vi "Start Water Draw Test Sequence SM.vi"(0 "Degree Setting":dbl=58.0, 1 "Equipment":T3={"COM Port"="COM1", "MW100"="MW100", "AG34970"="A-34972A", "WT500"="WT500"}, 2 "Semiphore":T2, 5 "Flow rate setting":dbl=3.0, 7 "Temp Band(+/- F)":dbl=50.0, 11 "Error In":errorcluster, 12 "Flow Chart Ref":refnum<vi>, 13 "Test Condition":T1(ring)=enum."DRK500,Station1,downspout") -> (4 "Downspout Flow":dbl=3.8899999999999997, 6 "Downspout Temp":dbl=76.8, 8 "Flow rate setting out":dbl=85.11482133995038, 15 "Error Out":errorcluster)   [LabVIEW 2009]
uses:
  EquipReferences.ctl
  Intellifaucet/Intellfaucet Mode.ctl
  ChannelSettings.ctl
panel:
  in  "Purge Min Time":i32=10000
  out "FlowSetTime":dbl
  out "FlowSetStartTime":dbl=3.0
  out "Settle Time Start":dbl format="%.2f"
  out "Purging":i32
  out "FlolwErrors":bool[](array[boolean])
  out "TempErrors":bool[](array[boolean])
  out "TempSet Time (sec)":dbl format="%.2f"
  out "error out":errorcluster
  in  "Sample Period(mS)":u32=500
  in  "Steady State Persist Time(mS)":u32=5000
  in  "Flow Adjust Time (3s)":dbl=3.0
  in  "Flow SettleTimeLimit(S)":dbl=300.0
  out "Downspout Flow Chart":dbl(graph)=3.8899999999999997
  out "Current State":string="Flow Settle"
  out "Downspout Temp Chart":dbl(graph)=76.8
  out "-E":dbl=54.11
  in  "Proportional Control Adjust Rate":dbl=0.1
  in  "Temp SettleTimeLimit(S)":dbl=20.0
  in  "Flow Band (+/-GPM)":dbl=0.25
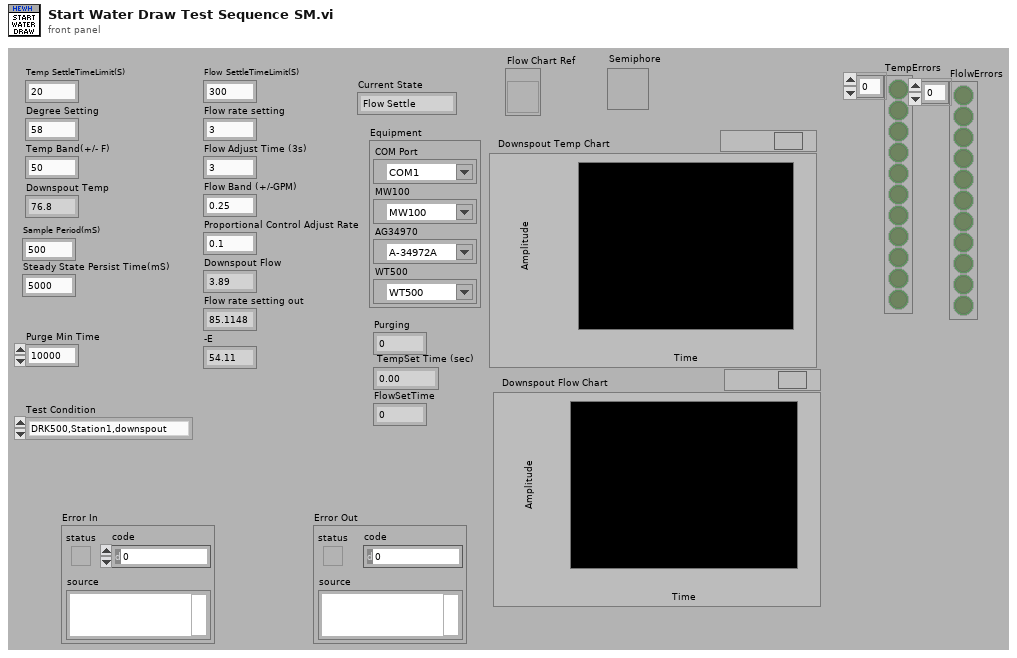
[diagram p1: front panel]
types:
  T1 = enum16{"DRK500,Station1", "DRK375,Lab", "SRK500,Station1,5GPM FR", "DRK500,Station1,downspout"}
  T2 = typedef "Semaphore RefNum" = refnum<k1>
  T3 = typedef "EquipReferences.ctl" = cluster{"COM Port":refnum<visa-resource-name>, "MW100":refnum<visa-resource-name>, "AG34970":refnum<visa-resource-name>, "WT500":refnum<visa-resource-name>}
  T4 = typedef "Intellfaucet Mode.ctl" = enum16{"Adjust Temp", "Adjust Flow", "Start Flow", "Stop Flow"}
  T5 = typedef "ChannelSettings.ctl" = u32
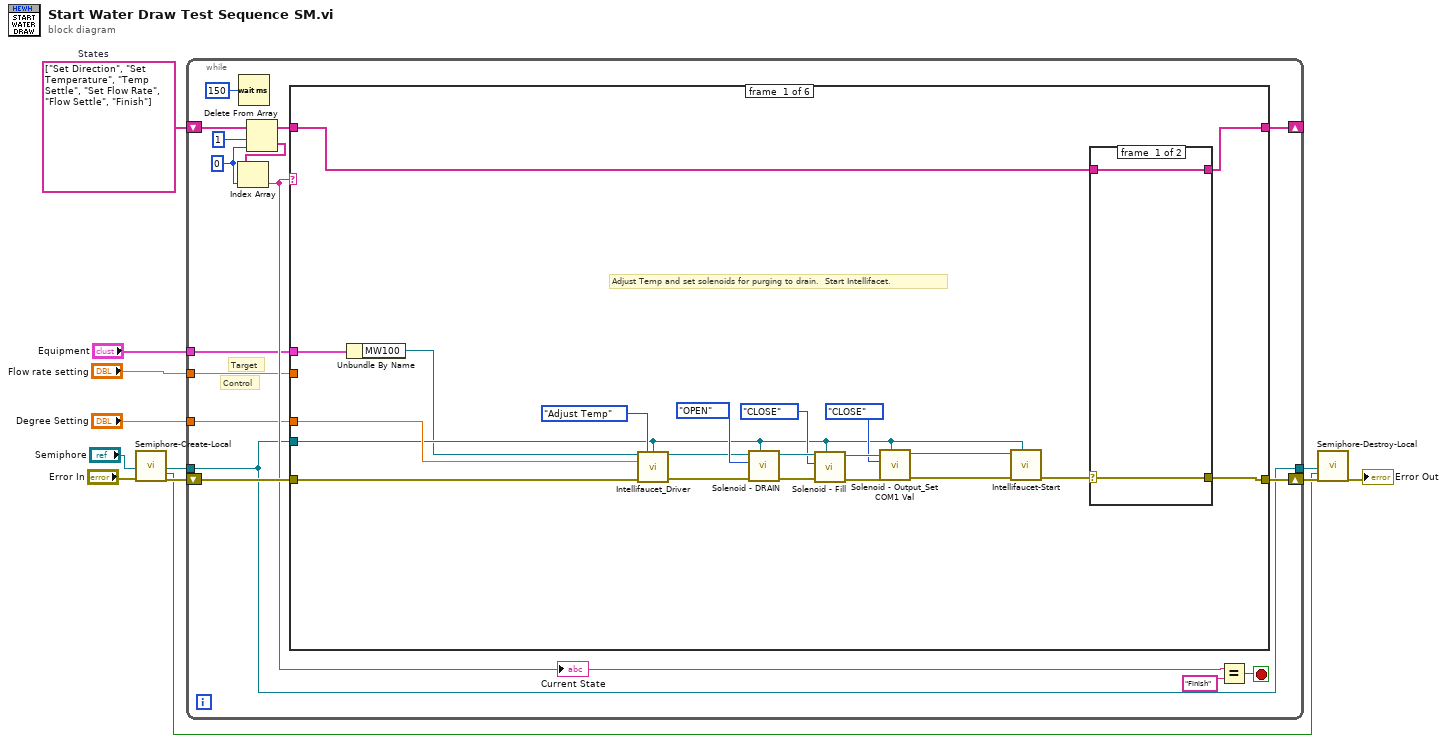
[diagram p0: block diagram]
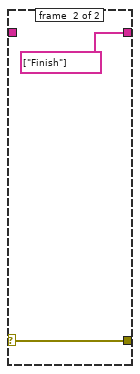
[diagram p2: hidden frame]
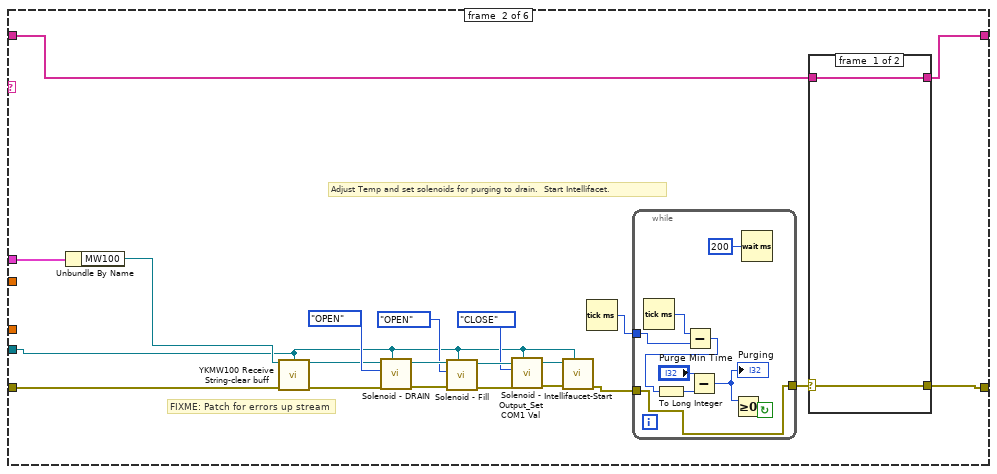
[diagram p3: hidden frame]
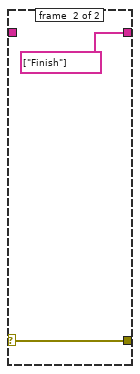
[diagram p4: hidden frame]
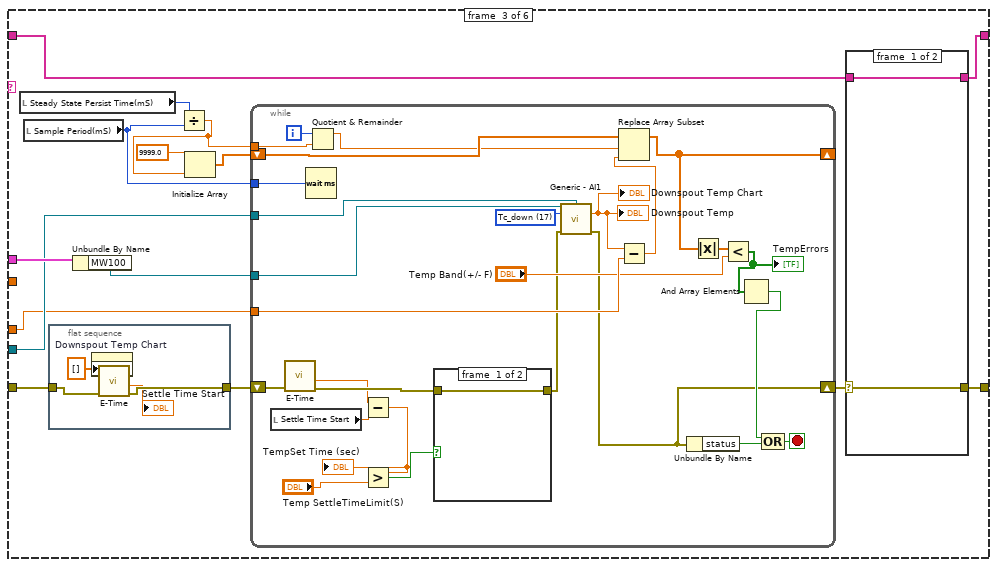
[diagram p5: hidden frame]
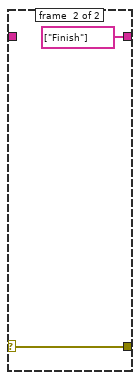
[diagram p6: hidden frame]
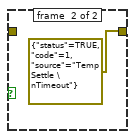
[diagram p7: hidden frame]
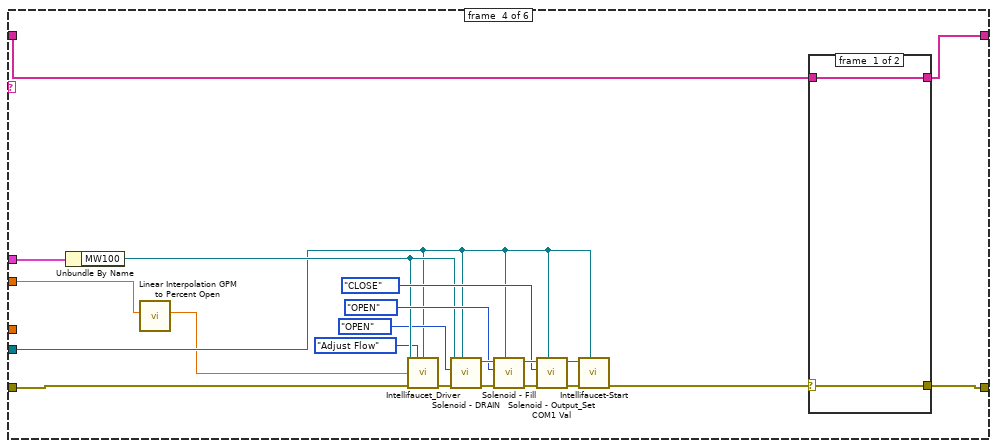
[diagram p8: hidden frame]
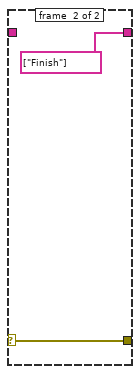
[diagram p9: hidden frame]
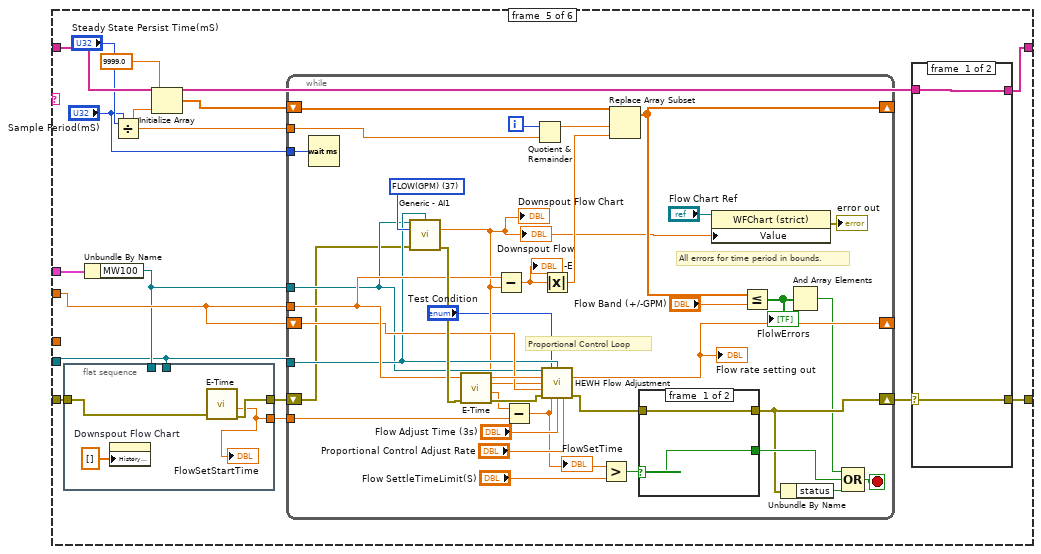
[diagram p10: hidden frame]
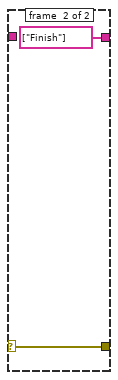
[diagram p11: hidden frame]
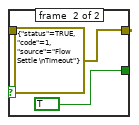
[diagram p12: hidden frame]
diagram:
  w12 = string[] ["Set Direction", "Set Temperature", "Temp Settle", "Set Flow Rate", "Flow Settle", "Finish"]  # States
  n1 = call "Semiphore-Create-Local.vi"("Semiphore"="Semiphore", "error in (no error)"="Error In") -> ("semaphore"=w2:T2, "Local?"=w3:bool, "error out"=w6:errorcluster)  [unwired: 15 in]
  n2 = while {
    shift-right: [w24] -> _
    shift-left: w12 -> [w28]
    shift-right: [w21] -> w5
    shift-left: w6 -> [w20]
    tunnel: "Equipment" -> [w16]
    tunnel: "Degree Setting" -> [w15]
    tunnel: "Flow rate setting" -> [w14]
    tunnel: w2 -> [w13]
    tunnel: [w13] -> w1
    stop <- w19 stop-if-true
    w25 = 0 ("index")
    # "Control"
    # "Target"
    n3 = Wait (ms)(milliseconds to wait=u32 150) -> ()  [unwired: 1 out]
    n4 = Delete From Array(array=w28, length=1, index=w25) -> (deleted portion=w26:string[], array with subset deleted=w23:string[])
    n5 = Index Array(array=w26, index=w25) -> (element=w18:string)
    "Current State" <- w18
    n6 = case shown="\"Flow Settle\"" w18 {
      tunnel: [w39 w72 w99 w150 w178 w232] -> w24
      tunnel: w23 -> [w40 w73 w100 w151 w179 w231]
      tunnel: [w37 w71 w97 w148 w176 w230] -> w21
      tunnel: w20 -> [w35 w58 w94 w146 w174 w229]
      tunnel: w16 -> [w49 w74 w102 w160 w180 _]
      tunnel: w15 -> [w34 _ w93 _ _ _]
      tunnel: w14 -> [_ _ _ w141 w173 _]
      tunnel: w13 -> [w31 w54 w96 w143 w166 _]
      frame #0 {
        # "Adjust Temp and set solenoids for purging to drain.  Start Intellifacet."
        n7 = Unbundle By Name(w49) -> ("MW100"=w30:refnum<visa-resource-name>)
        n8 = call "Intellifaucet_Driver.vi"("VISA session"=w30, "Mode"=Intellfaucet_Mode."Adjust Temp", "Semiphore"=w31, "Temperature(F)"=w34, "Error In"=w35) -> ("VISA session out"=w29:refnum<visa-resource-name>, "Error Out"=w36:errorcluster)  [unwired: 9 in]
        n9 = call "Solenoid - DRAIN.vi"("Semiphore"=w31, "Error In"=w36, "VALVE OPEN CLOSE"=enum8{"OPEN", "CLOSE"}."OPEN", "VISA session"=w29) -> ("Error Out"=w48:errorcluster, "dup VISA session"=w47:refnum<visa-resource-name>)  [unwired: 6 in]
        n10 = call "Solenoid - Fill.vi"("Semiphore"=w31, "Error In"=w48, "VALVE OPEN CLOSE"=enum8{"OPEN", "CLOSE"}."CLOSE" ("OPEN CLOSE"), "VISA session"=w47) -> ("Error Out"=w45:errorcluster, "dup VISA session"=w44:refnum<visa-resource-name>)  [unwired: 6 in]
        n11 = call "Solenoid - Output_Set COM1 Val.vi"("Semiphore"=w31, "Error In"=w45, "OPEN CLOSE"=enum8{"CLOSE", "OPEN"}."CLOSE", "VISA session"=w44) -> ("Error Out"=w42:errorcluster, "dup VISA session"=w41:refnum<visa-resource-name>)  [unwired: 6 in]
        n12 = call "Intellifaucet-Start.vi"("Semiphore"=w31, "Error In"=w42, "VISA session"=w41) -> ("Error Out"=w38:errorcluster)  [unwired: 7 in, 1 out]
        n13 = case shown="No Error" w38 {
          selector: w38 -> [w50 w53]
          tunnel: [w51 string[] ["Finish"] ("States")] -> w39
          tunnel: w40 -> [w51 _]
          tunnel: [w50 w53] -> w37
          frame #0 {
          }
          frame #1 {
          }
        }
      }
      frame #1 {
        # "FIXME: Patch for errors up stream"
        # "Adjust Temp and set solenoids for purging to drain.  Start Intellifacet."
        n14 = Unbundle By Name(w74) -> ("MW100"=w55:refnum<visa-resource-name>)
        n15 = call "YKMW100 Receive String-clear buff.vi"("VISA session"=w55, "Semiphore"=w54, "error in (no error)"=w58) -> ("dup VISA session"=w56:refnum<visa-resource-name>, "error out"=w57:errorcluster)  [unwired: 10 in, 1 out]
        n16 = call "Solenoid - DRAIN.vi"("Semiphore"=w54, "Error In"=w57, "VALVE OPEN CLOSE"=enum8{"OPEN", "CLOSE"}."OPEN", "VISA session"=w56) -> ("Error Out"=w68:errorcluster, "dup VISA session"=w67:refnum<visa-resource-name>)  [unwired: 6 in]
        n17 = call "Solenoid - Fill.vi"("Semiphore"=w54, "Error In"=w68, "VALVE OPEN CLOSE"=enum8{"OPEN", "CLOSE"}."OPEN" ("OPEN CLOSE"), "VISA session"=w67) -> ("Error Out"=w65:errorcluster, "dup VISA session"=w64:refnum<visa-resource-name>)  [unwired: 6 in]
        n18 = call "Solenoid - Output_Set COM1 Val.vi"("Semiphore"=w54, "Error In"=w65, "OPEN CLOSE"=enum8{"CLOSE", "OPEN"}."CLOSE", "VISA session"=w64) -> ("Error Out"=w61:errorcluster, "dup VISA session"=w59:refnum<visa-resource-name>)  [unwired: 6 in]
        n19 = call "Intellifaucet-Start.vi"("Semiphore"=w54, "Error In"=w61, "VISA session"=w59) -> ("Error Out"=w60:errorcluster)  [unwired: 7 in, 1 out]
        n20 = Tick Count (ms)() -> (millisecond timer value=w69:u32)
        n21 = while {
          tunnel: w60 -> [w77]
          tunnel: [w77] -> w70
          tunnel: w69 -> [w83]
          stop <- w80 continue-if-true
          n22 = Tick Count (ms)() -> (millisecond timer value=w82:u32)
          n23 = Subtract(x=w82, y=w83) -> (x-y=w76:u32)
          n24 = To Long Integer(number=w76) -> (32bit integer=w75:i32)
          n25 = Subtract(x="Purge Min Time", y=w75) -> (x-y=w79:i32)
          "Purging" <- w79
          n26 = Greater Or Equal To 0?(x=w79) -> (x >= 0?=w80:bool)
          n27 = Wait (ms)(milliseconds to wait=u32 200) -> ()  [unwired: 1 out]
        }
        n28 = case shown="Error" w70 {
          selector: w70 -> [w84 w87]
          tunnel: [w85 string[] ["Finish"] ("States")] -> w72
          tunnel: w73 -> [w85 _]
          tunnel: [w84 w87] -> w71
          frame #0 {
          }
          frame #1 {
          }
        }
      }
      frame #2 {
        n29 = local read "Steady State Persist Time(mS)"() -> (w92:u32)
        n30 = local read "Sample Period(mS)"() -> (w88:u32)
        n31 = flat-sequence {
          tunnel: [w105] -> w95
          tunnel: w94 -> [w104]
          frame #0 {
            n32 = property on="Downspout Temp Chart" class="WFChart (strict)"("History Data"=dbl[] []) -> ()  [unwired: 2 in, 2 out]
            n33 = call "E-Time.vi"("error in (no error)"=w104) -> ("error out"=w105:errorcluster, "Elapsed Time (sec)"=→"Settle Time Start":dbl)  [unwired: 8 in, 1 out]
          }
        }
        n34 = Unbundle By Name(w102) -> ("MW100"=w101:refnum<visa-resource-name>)
        n35 = Divide(x=w92, y=w88) -> (x/y=w90:dbl)
        n36 = Initialize Array(9999.0 ("element"), w90) -> (w89:dbl[])
        n37 = while {
          tunnel: w101 -> [w135]
          tunnel: w93 -> [w128]
          shift-right: [w114] -> w98
          shift-left: w95 -> [w118]
          tunnel: w96 -> [w133]
          tunnel: w90 -> [w130]
          shift-right: [w124] -> _
          shift-left: w89 -> [w129]
          tunnel: w88 -> [w119]
          i -> [w131]
          stop <- w137 stop-if-true
          w134 = T5 17 items=["4-20_OUT", "Pres_HI1", "Pres_HI2", "Pres_LOW", "Pres_PIN", "HEATER_TOP", "HEATER_BOT", "T_Shell", "FLOWMETER", "WATT_SENSE", "WH_TICK", "Tc_1", "Tc_2", "Tc_3", "Tc_4", "Tc_5", "Tc_6", "Tc_down", "T_Shell_2", "T_Shell_3", "T_Shell_4", "RTD_IN", "RTD_OUT", "RTD_AMB", "INTF_TEMPFLO", "INTF_READY", "INTF_START", "INTF_STOP", "DRM_LOW", "DRM_HIGH", "PWR_MAIN", "VLV_DUMP", "VLV_OUT", "VLV_IN", "WATT_HOURS", "FLOW(SAMPLE)", "GALLONS", "FLOW(GPM)"] ("Channel_Enum")
          n38 = local read "Settle Time Start"() -> (w113:dbl)
          n39 = call "E-Time.vi"("error in (no error)"=w118) -> ("error out"=w117:errorcluster, "Elapsed Time (sec)"=w112:dbl)  [unwired: 8 in, 1 out]
          n40 = Wait (ms)(milliseconds to wait=w119) -> ()  [unwired: 1 out]
          n41 = Quotient & Remainder(x=w131, y=w130) -> (x-y*floor(x/y)=w126:dbl)  [unwired: 1 out]
          n42 = Subtract(x=w112, y=w113) -> (x-y=w111:dbl)
          "TempSet Time (sec)" <- w111
          n43 = Greater?(x=w111, y="Temp SettleTimeLimit(S)") -> (0:w136:bool)
          n44 = case shown="True" w136 {
            tunnel: w117 -> [w138 _]
            tunnel: [w138 errorcluster {"status"=TRUE, "code"=1, "source"="Temp Settle \nTimeout"} ("Error In 2")] -> w116
            frame #0 {
            }
            frame #1 {
            }
          }
          n45 = call "Generic - AI1.vi"("MW100"=w135, "Semiphore"=w133, "Channel_Enum"=w134, "Error In"=w116) -> ("Value"=w127:dbl, "Error Out"=w114:errorcluster)  [unwired: 9 in, 1 out]
          "Downspout Temp" <- w127
          "Downspout Temp Chart" <- w127
          n46 = Subtract(x=w127, y=w128) -> (x-y=w125:dbl)
          n47 = Replace Array Subset(array=w129, new element=w125, index=w126) -> (w124:dbl[])
          n48 = Unbundle By Name(w114) -> ("status"=w115:bool)
          n49 = Absolute Value(x=w124) -> (abs(x)=w123:dbl[])
          n50 = Less?(x=w123, y="Temp Band(+/- F)") -> (x < y?=w121:bool[])
          "TempErrors" <- w121
          n51 = And Array Elements(Boolean array=w121) -> (logical AND=w120:bool)
          n52 = Compound Arithmetic op=OR(w120, w115) -> (w137:bool)
        }
        n53 = case shown="Error" w98 {
          selector: w98 -> [w107 w110]
          tunnel: [w108 string[] ["Finish"] ("States")] -> w99
          tunnel: w100 -> [w108 _]
          tunnel: [w107 w110] -> w97
          frame #0 {
          }
          frame #1 {
          }
        }
      }
      frame #3 {
        n54 = Unbundle By Name(w160) -> ("MW100"=w145:refnum<visa-resource-name>)
        n55 = call "Linear Interpolation GPM to Percent Open.vi"("Input (GPM,Percent)"=w141) -> ("Output (Percent,GPM)"=w140:dbl)  [unwired: 10 in]
        n56 = call "Intellifaucet_Driver.vi"("VISA session"=w145, "Mode"=Intellfaucet_Mode."Adjust Flow", "Semiphore"=w143, "Percent Flow"=w140, "Error In"=w146) -> ("Error Out"=w147:errorcluster)  [unwired: 9 in, 1 out]
        n57 = call "Solenoid - DRAIN.vi"("Semiphore"=w143, "Error In"=w147, "VALVE OPEN CLOSE"=enum8{"OPEN", "CLOSE"}."OPEN", "VISA session"=w145) -> ("Error Out"=w159:errorcluster, "dup VISA session"=w158:refnum<visa-resource-name>)  [unwired: 6 in]
        n58 = call "Solenoid - Fill.vi"("Semiphore"=w143, "Error In"=w159, "VALVE OPEN CLOSE"=enum8{"OPEN", "CLOSE"}."OPEN" ("OPEN CLOSE"), "VISA session"=w158) -> ("Error Out"=w156:errorcluster, "dup VISA session"=w155:refnum<visa-resource-name>)  [unwired: 6 in]
        n59 = call "Solenoid - Output_Set COM1 Val.vi"("Semiphore"=w143, "Error In"=w156, "OPEN CLOSE"=enum8{"CLOSE", "OPEN"}."CLOSE", "VISA session"=w155) -> ("Error Out"=w153:errorcluster, "dup VISA session"=w152:refnum<visa-resource-name>)  [unwired: 6 in]
        n60 = call "Intellifaucet-Start.vi"("Semiphore"=w143, "Error In"=w153, "VISA session"=w152) -> ("Error Out"=w149:errorcluster)  [unwired: 7 in, 1 out]
        n61 = case shown="Error" w149 {
          selector: w149 -> [w161 w164]
          tunnel: [w162 string[] ["Finish"] ("States")] -> w150
          tunnel: w151 -> [w162 _]
          tunnel: [w161 w164] -> w148
          frame #0 {
          }
          frame #1 {
          }
        }
      }
      frame #4 {
        n62 = flat-sequence {
          tunnel: [w183] -> w175
          tunnel: w174 -> [w181]
          tunnel: w167 -> [_]
          tunnel: w166 -> [_]
          tunnel: [w182] -> w165
          frame #0 {
            n63 = property on="Downspout Flow Chart" class="WFChart (strict)"("History Data"=dbl[] []) -> ()  [unwired: 2 in, 2 out]
            n64 = call "E-Time.vi"("error in (no error)"=w181) -> ("error out"=w183:errorcluster, "Elapsed Time (sec)"=w182:dbl)  [unwired: 8 in, 1 out]
            "FlowSetStartTime" <- w182
          }
        }
        n65 = Unbundle By Name(w180) -> ("MW100"=w167:refnum<visa-resource-name>)
        n66 = Divide(x="Steady State Persist Time(mS)", y="Sample Period(mS)") -> (x/y=w170:dbl)
        n67 = Initialize Array(9999.0 ("element"), w170) -> (w169:dbl[])
        n68 = while {
          tunnel: w167 -> [w195]
          shift-right: [w217] -> w177
          shift-left: w175 -> [w190]
          tunnel: w173 -> [w215]
          shift-right: [w210] -> _
          shift-left: w173 -> [w214]
          tunnel: w166 -> [w196]
          tunnel: w170 -> [w207]
          tunnel: "Sample Period(mS)" -> [w204]
          shift-right: [w200] -> _
          shift-left: w169 -> [w205]
          tunnel: w165 -> [w192]
          i -> [w208]
          stop <- w224 stop-if-true
          w197 = T5 37 items=["4-20_OUT", "Pres_HI1", "Pres_HI2", "Pres_LOW", "Pres_PIN", "HEATER_TOP", "HEATER_BOT", "T_Shell", "FLOWMETER", "WATT_SENSE", "WH_TICK", "Tc_1", "Tc_2", "Tc_3", "Tc_4", "Tc_5", "Tc_6", "Tc_down", "T_Shell_2", "T_Shell_3", "T_Shell_4", "RTD_IN", "RTD_OUT", "RTD_AMB", "INTF_TEMPFLO", "INTF_READY", "INTF_START", "INTF_STOP", "DRM_LOW", "DRM_HIGH", "PWR_MAIN", "VLV_DUMP", "VLV_OUT", "VLV_IN", "WATT_HOURS", "FLOW(SAMPLE)", "GALLONS", "FLOW(GPM)"] ("Channel_Enum")
          # "All errors for time period in bounds."
          # "Proportional Control Loop"
          n69 = Wait (ms)(milliseconds to wait=w204) -> ()  [unwired: 1 out]
          n70 = call "Generic - AI1.vi"("MW100"=w195, "Semiphore"=w196, "Channel_Enum"=w197, "Error In"=w190) -> ("Value"=w194:dbl, "Error Out"=w216:errorcluster)  [unwired: 9 in, 1 out]
          "Downspout Flow" <- w194
          "Downspout Flow Chart" <- w194
          n71 = call "E-Time.vi"("error in (no error)"=w216) -> ("error out"=w213:errorcluster, "Elapsed Time (sec)"=w193:dbl)  [unwired: 8 in, 1 out]
          n72 = Subtract(x=w215, y=w194) -> (x-y=w220:dbl)
          "-E" <- w220
          n73 = Subtract(x=w193, y=w192) -> (x-y=w191:dbl)
          "FlowSetTime" <- w191
          n74 = Quotient & Remainder(x=w208, y=w207) -> (x-y*floor(x/y)=w206:dbl)  [unwired: 1 out]
          n75 = Absolute Value(x=w220) -> (abs(x)=w203:dbl)
          n76 = call "HEWH Flow Adjustment.vi"("VISA session"=w195, "Test Condition"="Test Condition", "Semiphore"=w196, "GPM Target(3)"=w215, "GPM reading"=w194, "Flow rate setting In"=w214, "Error In"=w213, "Elapsed Time (sec)"=w191, "Flow Adjust Time (3s)"="Flow Adjust Time (3s)", "K(0.1)"="Proportional Control Adjust Rate") -> ("Flow rate setting Out"=w210:dbl, "Error Out"=w212:errorcluster)  [unwired: 3 in, 1 out]
          "Flow rate setting out" <- w210
          n77 = Greater?(x=w191, y="Flow SettleTimeLimit(S)") -> (0:w222:bool)
          n78 = Replace Array Subset(array=w205, new element=w203, index=w206) -> (w200:dbl[])
          n79 = case shown="True" w222 {
            selector: w222 -> [w226 _]
            tunnel: w212 -> [w225 _]
            tunnel: [w225 errorcluster {"status"=TRUE, "code"=1, "source"="Flow Settle \nTimeout"} ("Error In 2")] -> w217
            tunnel: [w226 TRUE] -> w223
            frame #0 {
            }
            frame #1 {
            }
          }
          n80 = property on="Property Node" class="WFChart (strict)"(reference="Flow Chart Ref", "Value"=w194) -> (error out=→"error out":errorcluster)  [unwired: 1 in, 1 out]
          n81 = Less Or Equal?(x=w200, y="Flow Band (+/-GPM)") -> (x <= y?=w202:bool[])
          "FlolwErrors" <- w202
          n82 = Unbundle By Name(w217) -> ("status"=w218:bool)
          n83 = And Array Elements(Boolean array=w202) -> (logical AND=w201:bool)
          n84 = Compound Arithmetic op=OR(w201, w223, w218) -> (w224:bool)
        }
        n85 = case shown="Error" w177 {
          selector: w177 -> [w185 w188]
          tunnel: [w186 string[] ["Finish"] ("States")] -> w178
          tunnel: w179 -> [w186 _]
          tunnel: [w185 w188] -> w176
          frame #0 {
          }
          frame #1 {
          }
        }
      }
      frame #5 {
        n86 = case shown="Error" w229 {
          selector: w229 -> [w233 w235]
          tunnel: [w234 w236] -> w232
          tunnel: w231 -> [w234 w236]
          tunnel: [w233 w235] -> w230
          frame #0 {
          }
          frame #1 {
          }
        }
      }
    }
    n87 = Equal?(x=w18, y="Finish") -> (x = y?=w19:bool)
  }
  n88 = call "Semiphore-Destroy-Local.vi"("Semiphore"=w1, "Local?"=w3, "error in (no error)"=w5) -> ("error out"=→"Error Out":errorcluster)  [unwired: 16 in]
